vi "Log.vi"(10 "Log Packet":T1, 11 "Buffered Log Sink in":refnum<class "Buffered Log Sink.lvclass">) -> (0 "error out":errorcluster, 3 "Buffered Log Sink out":refnum<class "Buffered Log Sink.lvclass">)   [LabVIEW 2019, in "Buffered Log Sink.lvclass"]
uses:
  <vilib>/gpm_packages/@cs/event-logger/Source/Buffered Log Sink/Buffered Log Sink.lvclass
  <vilib>/gpm_packages/@cs/event-logger/Source/Composed Log/Types/Log Packet.ctl
  <vilib>/gpm_packages/@cs/event-logger/Source/Composed Log/Types/Log Level.ctl
  <vilib>/gpm_packages/@cs/event-logger/Source/Buffered Log Sink/Buffered Log Sink.lvclass/Buffered Log Sink.ctl
  <vilib>/gpm_packages/@cs/event-logger/Source/Composed Log/Composed Log.lvlib
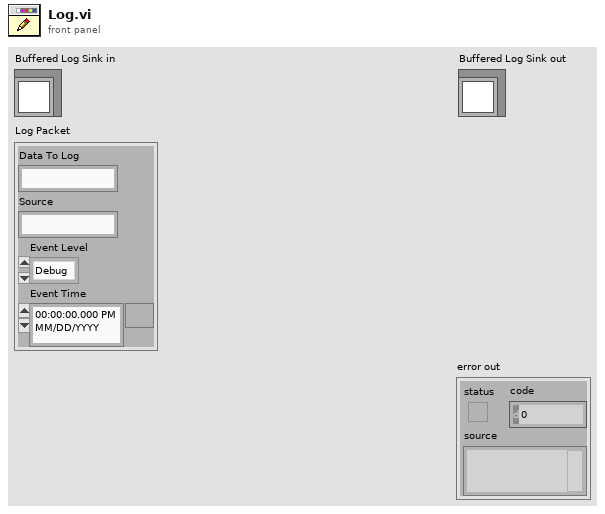
[diagram p1: front panel]
types:
  T1 = typedef "Composed Log.lvlib/Log Packet.ctl" = cluster{"Data To Log":string, "Source":string, "Event Level":T2, "Event Time":timestamp}
  T2 = typedef "Composed Log.lvlib/Log Level.ctl" = enum16{"Debug", "Info", "Warning", "Error", "Critical"}
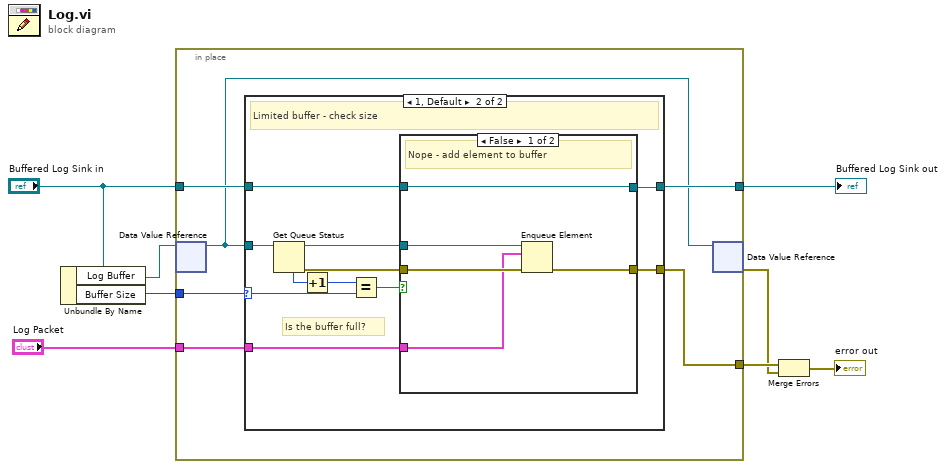
[diagram p0: block diagram]
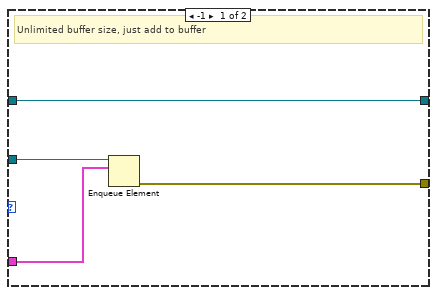
[diagram p2: hidden frame]
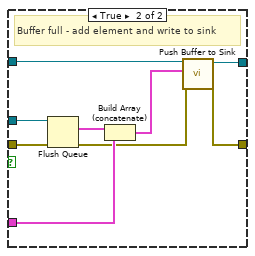
[diagram p3: hidden frame]
diagram:
  n1 = Unbundle By Name("Buffered Log Sink in") -> ("Log Buffer"=w3:refnum<data-value>, "Buffer Size"=w8:i32)
  n2 = in-place {
    in-place-border: w8 -> [w14]
    in-place-border: "Log Packet" -> [w13]
    in-place-border: [w12] -> w6
    in-place-border: "Buffered Log Sink in" -> [w11]
    in-place-border: [w10] -> w4
    n3 = in-place-dvr #1(w3) -> (w9:refnum<queue>)  [unwired: 1 out]
    n4 = case shown="1, Default" w14 {
      selector: w14 -> [_ w26]
      tunnel: w9 -> [w18 w29]
      tunnel: w13 -> [w17 w22]
      tunnel: [w16 w19] -> w12
      tunnel: w11 -> [w15 w25]
      tunnel: [w15 w20] -> w10
      frame -1 {
        # "Unlimited buffer size, just add to buffer"
        n5 = Enqueue Element(queue=w18, element=w17) -> (error out=w16:errorcluster)  [unwired: 2 in, 2 out]
      }
      frame 1, Default {
        # "Is the buffer full?"
        # "Limited buffer - check size"
        n6 = Get Queue Status(queue=w29) -> (queue out=w21:refnum<queue>, error out=w24:errorcluster, # elements in queue=w28:i32)  [unwired: 2 in, 5 out]
        n7 = Increment(x=w28) -> (x+1=w27:i32)
        n8 = Equal?(x=w27, y=w26) -> (x = y?=w23:bool)
        n9 = case shown="False" w23 {
          tunnel: w25 -> [w34 w39]
          tunnel: w24 -> [w33 w42]
          tunnel: w22 -> [w32 w40]
          tunnel: w21 -> [w30 w43]
          tunnel: [w34 w38] -> w20
          tunnel: [w31 w35] -> w19
          frame False {
            # "Nope - add element to buffer"
            n10 = Enqueue Element(queue=w30, element=w32, error in (no error)=w33) -> (error out=w31:errorcluster)  [unwired: 1 in, 2 out]
          }
          frame True {
            # "Buffer full - add element and write to sink"
            n11 = Flush Queue(queue=w43, error in (no error)=w42) -> (remaining elements=w41:T1[], error out=w36:errorcluster)  [unwired: 1 out]
            n12 = Build Array (concatenate)(w41, w40) -> (w37:T1[])
            n13 = call <vilib>:"Push Buffer to Sink.vi"("error in (no error)"=w36, "Log Events"=w37, "Buffered Log Sink in"=w39) -> ("error out"=w35:errorcluster, "Buffered Log Sink out"=w38:refnum<class "Buffered Log Sink.lvclass">)  [unwired: 7 in]
          }
        }
      }
    }
    n14 = in-place-dvr #1(w9) -> (w1:errorcluster)  [unwired: 1 out]
  }
  "Buffered Log Sink out" <- w4
  n15 = Merge Errors(w6, w1) -> (→"error out":errorcluster)
